vi "2 inputs loop.vi"() -> ()   [LabVIEW 2015]
doc: "This example VI shows how to convert string data elements to numeric elements so it can be graphed and displayed on an XY Graph."
uses:
  <instrlib>/Keithley 27XX/Public/Data/Read Multiple Direct.vi
  <instrlib>/Keithley 27XX/Keithley 27XX.lvlib
panel:
  in  "Pause/Continue":bool
  in  "stop":bool
  out "Numeric":i32
  out "concatenated string":string
  out "XY Graph":T1(graph)
  in  "file (use dialog)":path=path "C:/Users/Guest_2/Desktop/Zong Long/Data trial.txt"
  in  "Function (6: Temp)":u16(ring)=6 items=["DC Voltage", "AC Voltage", "DC Current", "AC Current", "Resistance", "Four-Wire Resistance", "Temperature (C)", "Frequency", "Period", "Continuity"]
  in  "Sample Count (10)":i32=10
  in  "Channel List (101)":string="101"
  in  "Serial Configuration":T2={"Baud Rate (9600)"=9600, "Flow Control (1: XON/XOFF)"=1, "Termination Char (0:CR)"=0} {"Termination Char (0:CR)" items=["CR", "LF", "CRLF (Do not use)", "LFCR (Do not use)"]; "Flow Control (1: XON/XOFF)" items=["None", "XON/XOFF", "RTS/CTS (2701 Only)", "XON/XOFF & RTS/CTS (2701 Only)"]; "Baud Rate (9600)" items=["300"=300, "600"=600, "1200"=1200, "2400"=2400, "4800"=4800, "9600"=9600, "19.2k"=19200, "38.4k (2701 Only)"=38400, "57.6k (2701 Only)"=57600, "115.2k (2701 Only)"=115200]}
  in  "Timeout (30000 milliseconds)":u32=30000
  in  "VISA resource name":refnum<visa-resource-name>="GPIB0::19::INSTR"
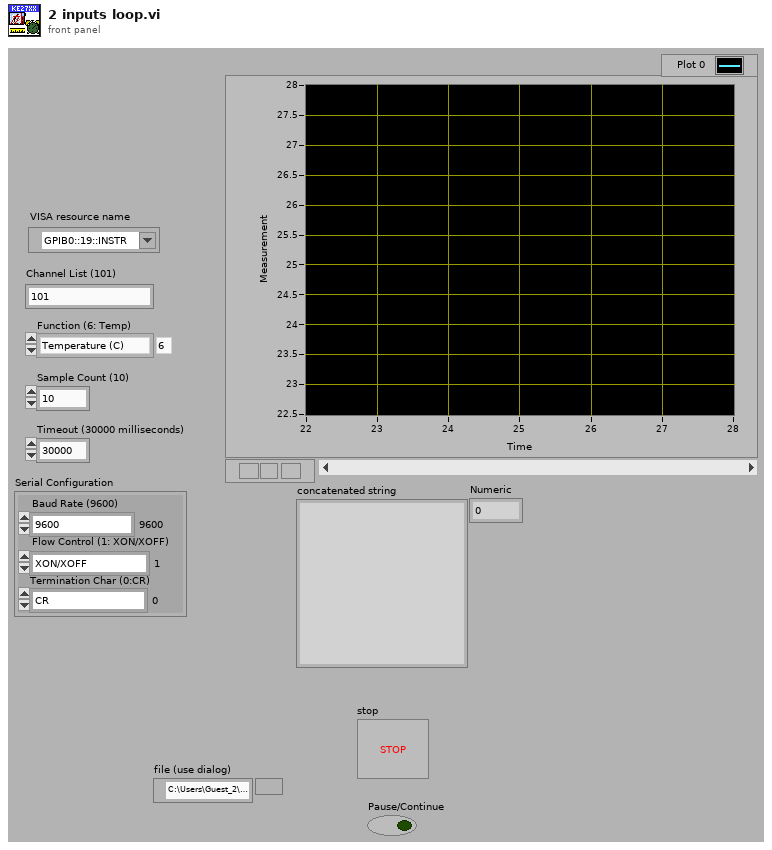
[diagram p1: front panel]
types:
  T1 = cluster{"Measurement Data":dbl[], "Converted Numeric Array":dbl[]}
  T2 = cluster{"Baud Rate (9600)":u32, "Flow Control (1: XON/XOFF)":u16, "Termination Char (0:CR)":u16}
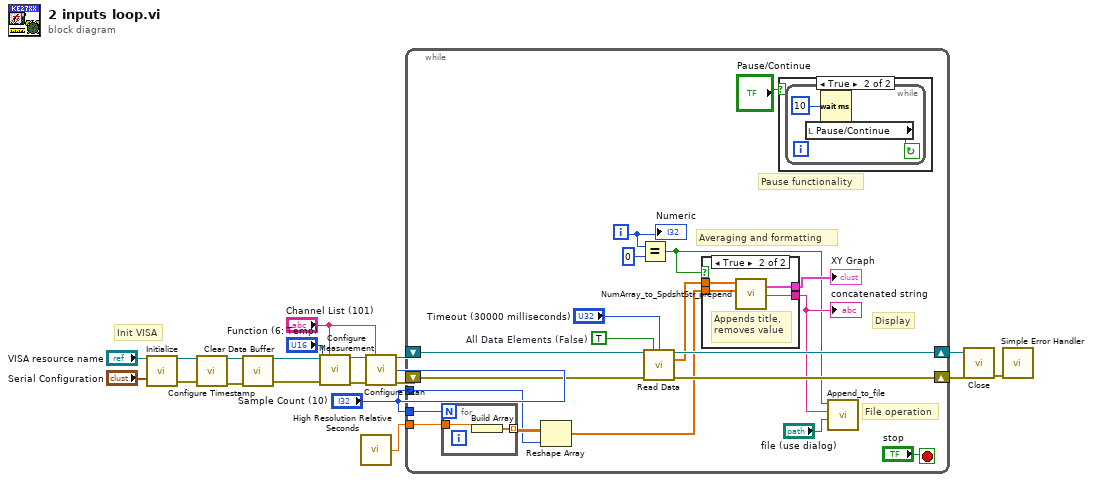
[diagram p0: block diagram]
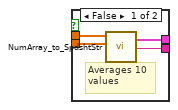
[diagram p3: hidden frame]
diagram:
  # "Init VISA"
  n1 = call <instrlib>:"Initialize.vi"("VISA resource name"="VISA resource name", "Serial Configuration"="Serial Configuration") -> ("VISA resource name out"=w16:refnum<visa-resource-name>, "error out"=w15:errorcluster)  [unwired: 12 in]
  n2 = call <instrlib>:"Configure Timestamp.vi"("VISA resource name"=w16, "error in (no error)"=w15) -> ("VISA resource name out"=w11:refnum<visa-resource-name>, "error out"=w10:errorcluster)  [unwired: 12 in]
  n3 = call <instrlib>:"Clear Data Buffer.vi"("VISA resource name"=w11, "error in (no error)"=w10) -> ("VISA resource name out"=w9:refnum<visa-resource-name>, "error out"=w12:errorcluster)  [unwired: 12 in]
  n4 = call <instrlib>:"Configure Measurement.vi"("VISA resource name"=w9, "Scan List (Empty)"="Channel List (101)", "Function (0: DC Voltage)"="Function (6: Temp)", "error in (no error)"=w12) -> ("VISA resource name out"=w8:refnum<visa-resource-name>, "error out"=w6:errorcluster)  [unwired: 10 in]
  n5 = call <vilib>:"High Resolution Relative Seconds.vi"() -> ("relative seconds"=w2:dbl)
  n6 = call <instrlib>:"Configure Scan.vi"("VISA resource name"=w8, "Channel List (101:110)"="Channel List (101)", "Sample Count (100)"="Sample Count (10)", "error in (no error)"=w6) -> ("VISA resource name out"=w4:refnum<visa-resource-name>, "error out"=w3:errorcluster)  [unwired: 10 in]
  n7 = while {
    shift-right: [w38] -> w13
    shift-left: w4 -> [w35]
    shift-right: [w39] -> w14
    shift-left: w3 -> [w34]
    tunnel: "Sample Count (10)" -> [w28]
    tunnel: w2 -> [w27]
    tunnel: "Sample Count (10)" -> [w25]
    i -> [w20]
    stop <- "stop" stop-if-true
    w37 = TRUE  # All Data Elements (False)
    # "Display"
    # "Averaging and formatting"
    # "File operation"
    # "Pause functionality"
    n8 = for {
      N: w28 -> [_]
      tunnel: w27 -> [w43]
      tunnel: [w42] -> w26 mode=indexing
      n9 = Build Array(w43) -> (w42:dbl[])
    }
    n10 = Reshape Array(w26, w25) -> (w24:dbl[])
    n11 = Equal?(x=w20, y=0) -> (x = y?=w22:bool)
    n12 = call-poly <instrlib>:"Read Data.vi"("VISA resource name"=w35, "All Data Elements (False)"=w37, "Timeout (30000 milliseconds)"="Timeout (30000 milliseconds)", "error in (no error)"=w34) -> ("VISA resource name out"=w38:refnum<visa-resource-name>, "Measurement Data"=w32:dbl[], "error out"=w39:errorcluster)  [unwired: 6 in, 3 out]
    n13 = case shown="True" w22 {
      tunnel: w32 -> [w47 w51]
      tunnel: w24 -> [w46 w50]
      tunnel: [w45 w48] -> w31
      tunnel: [w44 w49] -> w30
      frame False {
        # "Averages 10 \nvalues"
        n14 = call "NumArray_to_SpdshtStr.vi"("element 2"=w46, "element"=w47) -> ("concatenated string"=w44:string, "XY Graph"=w45:T1)  [unwired: 8 in]
      }
      frame True {
        # "Appends title,\nremoves value"
        n15 = call "NumArray_to_SpdshtStr_prepend.vi"("timestamp"=w50, "element"=w51) -> ("concatenated string"=w49:string, "XY Graph"=w48:T1)  [unwired: 8 in]
      }
    }
    "XY Graph" <- w31
    "concatenated string" <- w30
    n16 = case shown="True" "Pause/Continue" {
      frame False {
      }
      frame True {
        n17 = while {
          stop <- w41 continue-if-true
          n18 = local read "Pause/Continue"() -> (w41:bool)
          n19 = Wait (ms)(milliseconds to wait=u32 10) -> ()  [unwired: 1 out]
        }
      }
    }
    n20 = call "Append_to_file.vi"("file path (use dialog)"="file (use dialog)", "text"=w30, "Boolean"=w22) -> ()  [unwired: 8 in, 1 out]
    "Numeric" <- w20
  }
  n21 = call <instrlib>:"Close.vi"("VISA resource name"=w13, "error in (no error)"=w14) -> ("error out"=w17:errorcluster)  [unwired: 13 in]
  n22 = call <vilib>:"Simple Error Handler.vi"("error in (no error)"=w17) -> ()  [unwired: 4 in, 5 out]
